vi "GetNodeMenuOptions.vi"(0 "reference":refnum<class "ClassNode.lvclass">, 1 "MousePos":T1 {"y" format="%.2f"; "x" format="%.2f"}, 5 "error in (no error)":errorcluster) -> (14 "reference out":refnum<class "ClassNode.lvclass">, 15 "MenuOptions":string[](array[string]), 19 "error out":errorcluster)   [LabVIEW 2014, in "ClassNode.lvclass"]
doc: "Gets the menu option"
uses:
  <resource>/Framework/Providers/Open_GDS/UML/ClassNode_class/ClassNode.lvclass
  <resource>/Framework/Providers/Open_GDS/UML/General/Point/Point Point2D.ctl
  <resource>/Framework/Providers/Open_GDS/UML/RectangularNode_class/RectangularNode.lvclass
  <resource>/Framework/Providers/Open_GDS/UML/MultiLineString_class/MultiLineString.lvclass
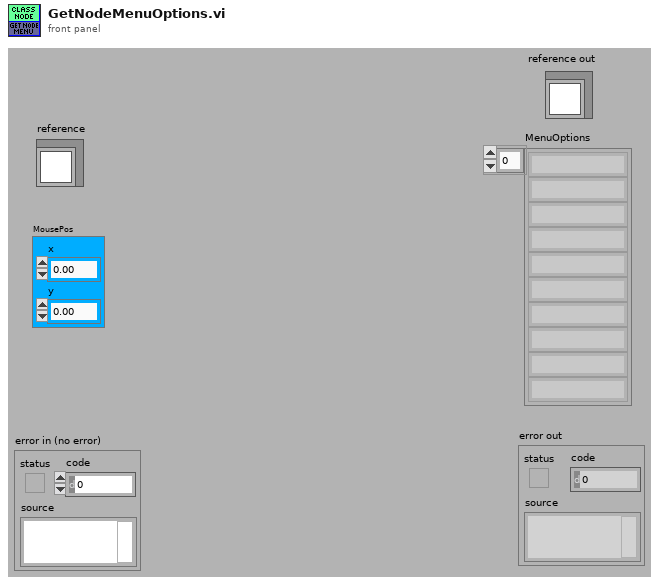
[diagram p1: front panel]
types:
  T1 = typedef "Point Point2D.ctl" = cluster{"x":dbl, "y":dbl}
  T2 = typedef "ClassNode.lvclass/ObjectAttributes.ctl" = cluster{"Base class":T3, "midHeight":dbl, "botHeight":dbl, "name":refnum<class "MultiLineString.lvclass">, "attributes":refnum<class "MultiLineString.lvclass">, "methods":refnum<class "MultiLineString.lvclass">, "DEFAULT_COMPARTMENT_HEIGHT":i32, "DEFAULT_WIDTH":i32, "DEFAULT_HEIGHT":i32, "showMethods":bool, "showAttributes":bool, "ClassPath":path}
  T3 = typedef "RectangularNode.lvclass/ObjectAttributes.ctl" = cluster{"Base class":T4, "bounds":T5}
  T4 = typedef "AbstractNode.lvclass/ObjectAttributes.ctl" = cluster{"parent":refnum<class "AbstractNode.lvclass">, "children":refnum<class "AbstractNode.lvclass">[], "Hidden":bool}
  T5 = typedef "Rectangle Rectangle2D.ctl" = cluster{"x":dbl, "y":dbl, "width":dbl, "height":dbl}
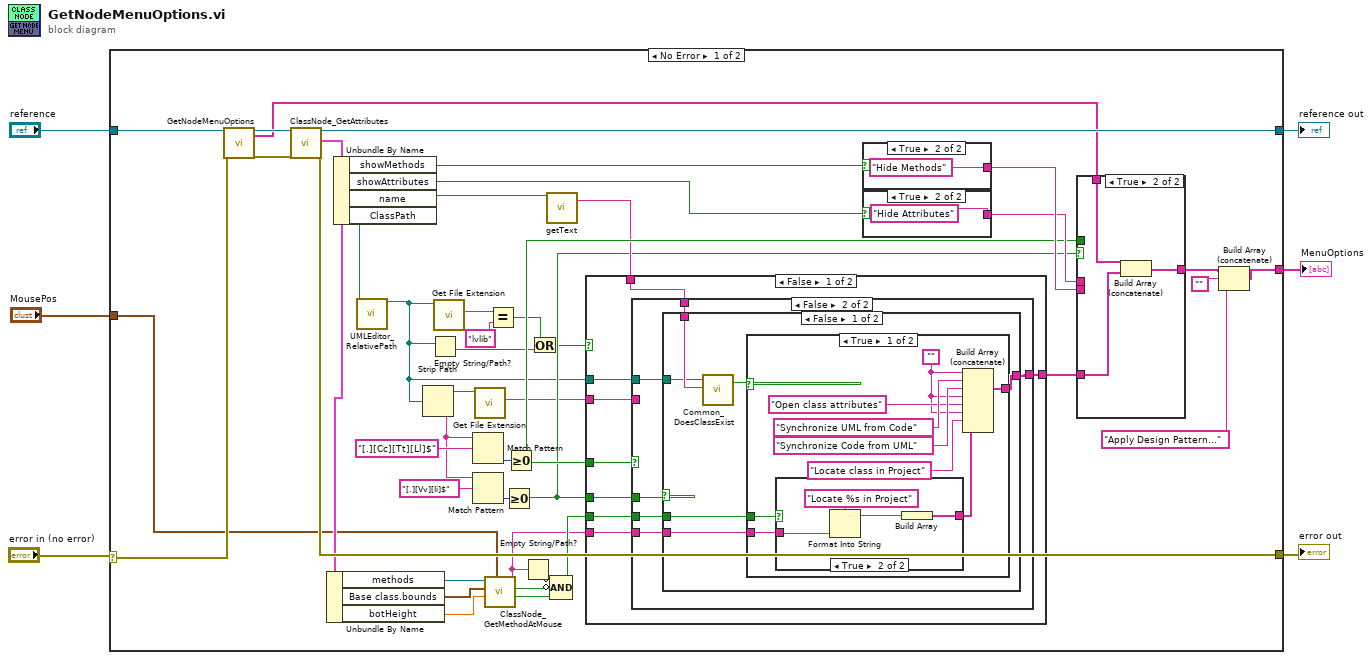
[diagram p0: block diagram]
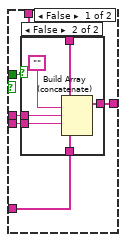
[diagram p2: hidden frame]
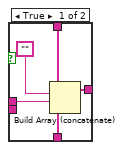
[diagram p3: hidden frame]
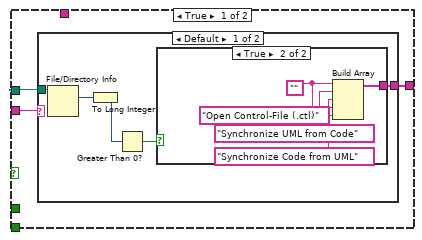
[diagram p4: hidden frame]
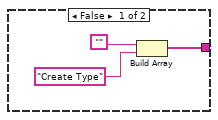
[diagram p5: hidden frame]
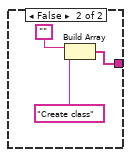
[diagram p8: hidden frame]
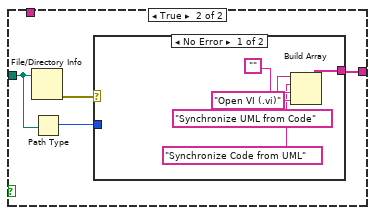
[diagram p9: hidden frame]
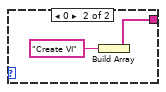
[diagram p11: hidden frame]
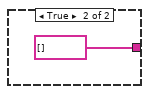
[diagram p12: hidden frame]
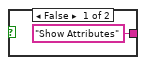
[diagram p13: hidden frame]
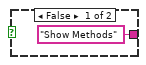
[diagram p14: hidden frame]
diagram:
  n1 = case shown="No Error" "error in (no error)" {
    selector: "error in (no error)" -> [w22 w141]
    tunnel: "reference" -> [w23 w142]
    tunnel: [w50 w141] -> w5
    tunnel: [w49 w142] -> w4
    tunnel: [w9 _] -> w2
    tunnel: "MousePos" -> [w18 _]
    frame No Error {
      n2 = call-parent "GetNodeMenuOptions.vi"("reference"=w23, "error in (no error)"=w22) -> ("reference out"=w25:refnum<class "ClassNode.lvclass">, "MenuOptions"=w24:string[], "error out"=w21:errorcluster)  [unwired: 15 in]
      n3 = call <resource>:"ClassNode_GetAttributes.vi"("reference in"=w25, "error in (no error)"=w21) -> ("reference out"=w49:refnum<class "ClassNode.lvclass">, "Attributes"=w20:T2, "error out"=w50:errorcluster)  [unwired: 15 out]
      n4 = Unbundle By Name(w20) -> ("methods"=w19:refnum<class "MultiLineString.lvclass">, "Base class.bounds"=w17:T5, "botHeight"=w16:dbl)
      n5 = Unbundle By Name(w20) -> ("showMethods"=w48:bool, "showAttributes"=w47:bool, "name"=w40:refnum<class "MultiLineString.lvclass">, "ClassPath"=w38:path)
      n6 = call <resource>:"UMLEditor_RelativePath.vi"("Path In"=w38) -> ("ConvertToAbsolutePath(If possible)"=w33:path)  [unwired: 1 in, 17 out]
      n7 = Strip Path(path=w33) -> (stripped path=w27:path, name=w37:string)
      n8 = Empty String/Path?(string/path=w33) -> (empty?=w29:bool)
      n9 = call <vilib>:"Get File Extension.vi"("file"=w33) -> ("lowercase file extension"=w32:string)  [unwired: 1 in, 9 out]
      n10 = Match Pattern(string=w37, regular expression="[.][Cc][Tt][Ll]$") -> (offset past match=w42:i32)  [unwired: 4 out]
      n11 = Match Pattern(string=w37, regular expression="[.][Vv][Ii]$") -> (offset past match=w35:i32)  [unwired: 4 out]
      n12 = call <vilib>:"Get File Extension.vi"("file"=w27) -> ("lowercase file extension"=w26:string)  [unwired: 1 in, 9 out]
      n13 = call <resource>:"ClassNode_GetMethodAtMouse.vi"("MousePos"=w18, "botHeight"=w16, "bounds"=w17, "methods"=w19) -> ("MethodSelected"=w14:bool, "NoMmethodsExists"=w15:bool, "MEthodName"=w11:string)  [unwired: 2 in, 1 out]
      n14 = Equal?(x=w32, y="lvlib") -> (x = y?=w28:bool)
      n15 = Greater Or Equal To 0?(x=w35) -> (x >= 0?=w34:bool)
      n16 = Greater Or Equal To 0?(x=w42) -> (x >= 0?=w41:bool)
      n17 = Empty String/Path?(string/path=w11) -> (empty?=w13:bool)
      n18 = Or(x=w28, y=w29) -> (x .or. y?=w30:bool)
      n19 = call-dynamic "getText.vi"("reference"=w40) -> ("text"=w39:string)  [unwired: 16 in, 2 out]
      n20 = Compound Arithmetic op=AND(invert w13, invert w15, w14) -> (w12:bool)
      n21 = case shown="False" w30 {
        tunnel: [w78 string[] []] -> w46
        tunnel: w41 -> [w77 _]
        tunnel: w33 -> [w76 _]
        tunnel: w39 -> [w75 _]
        tunnel: w34 -> [w74 _]
        tunnel: w26 -> [w73 _]
        tunnel: w12 -> [w72 _]
        tunnel: w11 -> [w71 _]
        frame False {
          n22 = case shown="False" w77 {
            tunnel: [w81 w100] -> w78
            tunnel: w76 -> [w80 w98]
            tunnel: w75 -> [_ w99]
            tunnel: w74 -> [_ w97]
            tunnel: w73 -> [w79 _]
            tunnel: w72 -> [_ w96]
            tunnel: w71 -> [_ w95]
            frame True {
              n23 = case shown="Default" w79 {
                tunnel: [w86 _] -> w81
                tunnel: w80 -> [w84 _]
                frame Default {
                  n24 = File/Directory Info(path=w84) -> (size=w82:i64)  [unwired: 1 in, 6 out]
                  n25 = To Long Integer(number=w82) -> (32bit integer=w85:i32)
                  n26 = Greater Than 0?(x=w85) -> (x > 0?=w83:bool)
                  n27 = case shown="True" w83 {
                    tunnel: [w88 w94] -> w86
                    frame False {
                      n28 = Build Array("", "Create Type" ("element")) -> (w88:string[])
                    }
                    frame True {
                      w91 = ""
                      n29 = Build Array(w91, "Synchronize UML from Code" ("element"), "Synchronize Code from UML" ("element"), w91, "Open Control-File (.ctl)" ("element")) -> (w94:string[])
                    }
                  }
                }
                frame "lvclass" {
                }
              }
            }
            frame False {
              n30 = case shown="False" w97 {
                tunnel: [w106 w126] -> w100
                tunnel: w99 -> [w105 _]
                tunnel: w98 -> [w103 w124]
                tunnel: w96 -> [w102 _]
                tunnel: w95 -> [w101 _]
                frame False {
                  n31 = call <resource>:"Common_DoesClassExist.vi"("ClassPath"=w103, "ClassName"=w105) -> ("ClassExists"=w104:bool)  [unwired: 17 out]
                  n32 = case shown="True" w104 {
                    tunnel: [w115 w122] -> w106
                    tunnel: w102 -> [w109 _]
                    tunnel: w101 -> [w108 _]
                    frame True {
                      w111 = ""
                      n33 = case shown="True" w109 {
                        tunnel: w108 -> [_ w119]
                        tunnel: [_ w116] -> w107
                        frame False {
                        }
                        frame True {
                          n34 = Format Into String(format string="Locate %s in Project" ("element"), w119) -> (resulting string=w117:string)  [unwired: 2 in, 1 out]
                          n35 = Build Array(w117) -> (w116:string[])
                        }
                      }
                      n36 = Build Array (concatenate)(w111, "Synchronize UML from Code" ("element"), "Synchronize Code from UML" ("element"), w111, "Open class attributes" ("element"), w111, "Locate class in Project" ("element"), w107) -> (w115:string[])
                    }
                    frame False {
                      n37 = Build Array("", "Create class" ("element")) -> (w122:string[])
                    }
                  }
                }
                frame True {
                  n38 = File/Directory Info(path=w124) -> (error out=w125:errorcluster)  [unwired: 1 in, 6 out]
                  n39 = Path Type(1:w124) -> (0:w123:i16)
                  n40 = case shown="No Error" w125 {
                    tunnel: [w131 w133] -> w126
                    tunnel: w123 -> [_ w132]
                    frame No Error {
                      n41 = Build Array("Synchronize UML from Code" ("element"), "Synchronize Code from UML" ("element"), "", "Open VI (.vi)" ("element")) -> (w131:string[])
                    }
                    frame Error {
                      n42 = case shown="Default" w132 {
                        tunnel: [_ w135] -> w133
                        frame Default {
                        }
                        frame 0 {
                          n43 = Build Array("Create VI" ("element")) -> (w135:string[])
                        }
                      }
                    }
                  }
                }
              }
            }
          }
        }
        frame True {
        }
      }
      n44 = case shown="True" w48 {
        tunnel: ["Show Methods" "Hide Methods"] -> w45
        frame False {
        }
        frame True {
        }
      }
      n45 = case shown="True" w47 {
        tunnel: ["Show Attributes" "Hide Attributes"] -> w44
        frame False {
        }
        frame True {
        }
      }
      n46 = case shown="True" w34 {
        tunnel: [w56 w70] -> w10
        tunnel: w46 -> [w55 w69]
        tunnel: w45 -> [w54 _]
        tunnel: w44 -> [w53 _]
        tunnel: w41 -> [w52 _]
        tunnel: w24 -> [w51 w68]
        frame False {
          n47 = case shown="False" w52 {
            tunnel: [w61 w67] -> w56
            tunnel: w55 -> [w58 w65]
            tunnel: w54 -> [_ w64]
            tunnel: w53 -> [w59 w63]
            tunnel: w51 -> [w57 w62]
            frame True {
              n48 = Build Array (concatenate)(w57, "", w59, w58) -> (w61:string[])
            }
            frame False {
              n49 = Build Array (concatenate)(w62, "", w63, w64, w65) -> (w67:string[])
            }
          }
        }
        frame True {
          n50 = Build Array (concatenate)(w68, w69) -> (w70:string[])
        }
      }
      n51 = Build Array (concatenate)(w10, "", "Apply Design Pattern..." ("element")) -> (w9:string[])
    }
    frame Error {
    }
  }
  "reference out" <- w4
  "error out" <- w5
  "MenuOptions" <- w2
